vi "Power Supply Global.vi"(0 "Closed Loop":bool, 2 "PS Global Mode":T1, 5 "PS Cmd":dbl min=0.0 max=20.0 format="%#.2f", 7 "PS Voltage":dbl, 9 "FreezePID":bool) -> (4 "Closed Loop OUT":bool, 6 "PS Cmd OUT":dbl, 8 "PS Voltage OUT":dbl, 10 "FreezePID OUT":bool)   [LabVIEW 2013]
uses:
  Controls/Power Supply Global Mode.ctl
panel:
  in  "Power Supply Cmd (V):":dbl min=0.0 max=20.0 format="%#.2f"
  in  "Closed Loop Voltage":bool
  out "FreezePID":bool
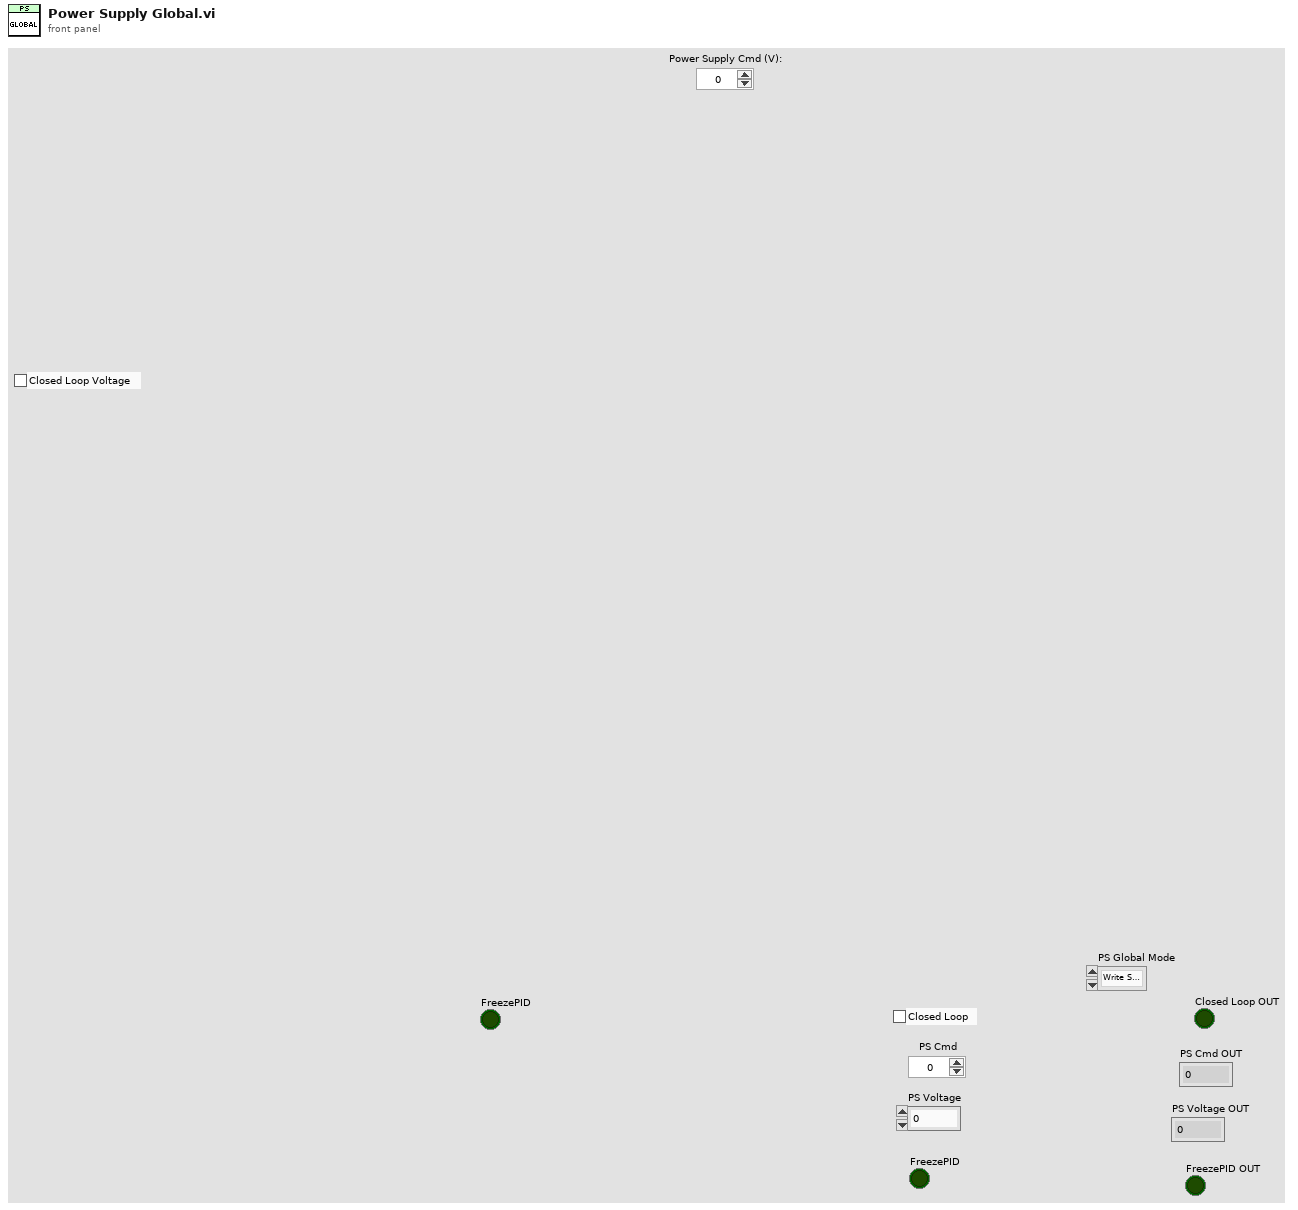
[diagram p1: front panel]
types:
  T1 = typedef "Power Supply Global Mode.ctl" = enum16{"Write Setpoint", "Write FreezePID", "Read"}
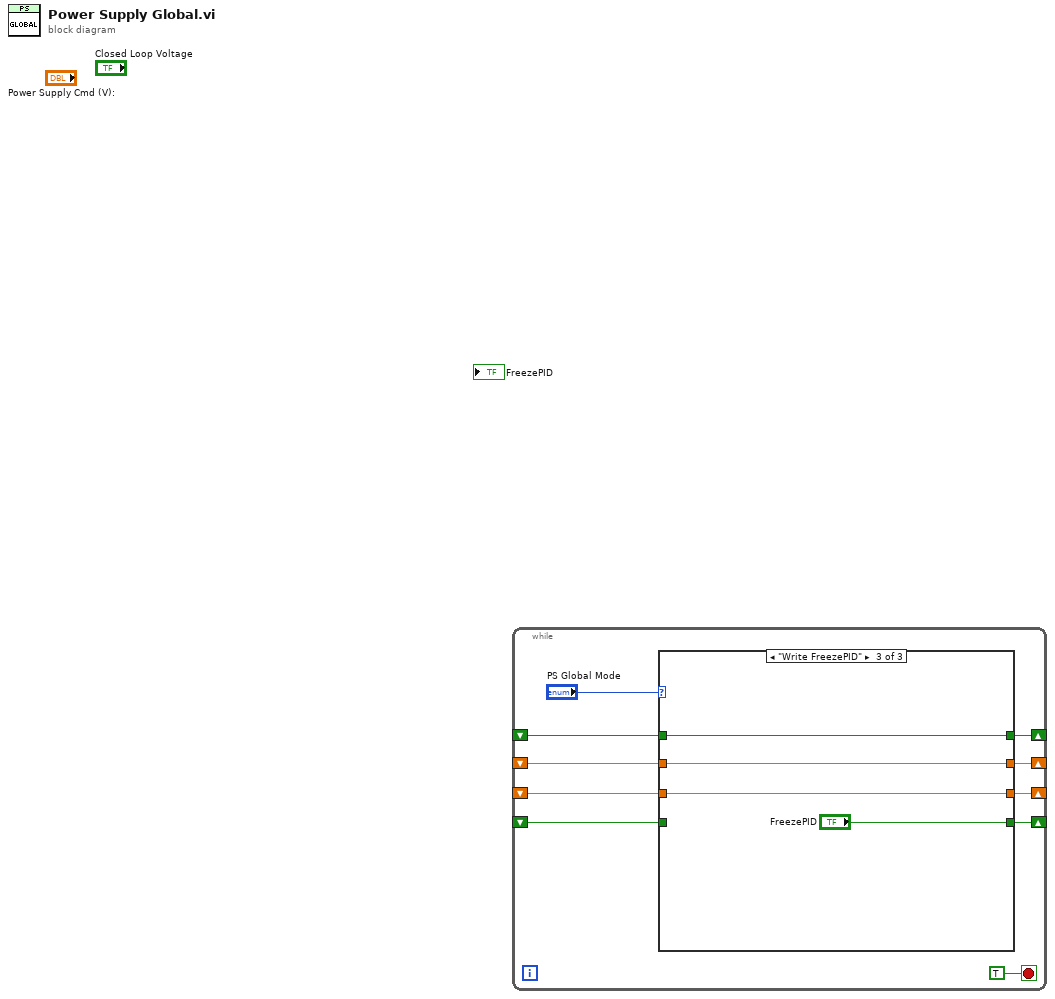
[diagram p0: block diagram]
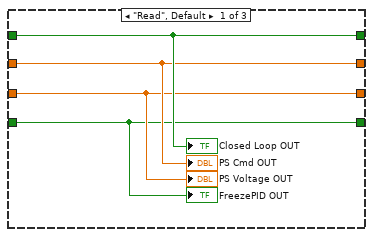
[diagram p2: hidden frame]
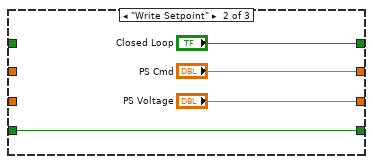
[diagram p3: hidden frame]
diagram:
  n1 = while {
    shift-right: [w9] -> _
    shift-left: _ -> [w5]
    shift-right: [w8] -> _
    shift-left: _ -> [w4]
    shift-right: [w7] -> _
    shift-left: _ -> [w3]
    shift-right: [w6] -> _
    shift-left: _ -> [w2]
    stop <- TRUE stop-if-true
    n2 = case shown="\"Write FreezePID\"" "PS Global Mode" {
      tunnel: [w14 "Closed Loop" w22] -> w9
      tunnel: [w13 "PS Cmd" w21] -> w8
      tunnel: [w12 "PS Voltage" w20] -> w7
      tunnel: [w11 w15 "FreezePID"] -> w6
      tunnel: w5 -> [w14 _ w22]
      tunnel: w4 -> [w13 _ w21]
      tunnel: w3 -> [w12 _ w20]
      tunnel: w2 -> [w11 w15 _]
      frame "Read", Default {
        "Closed Loop OUT" <- w14
        "PS Cmd OUT" <- w13
        "PS Voltage OUT" <- w12
        "FreezePID OUT" <- w11
      }
      frame "Write Setpoint" {
      }
      frame "Write FreezePID" {
      }
    }
  }
